vi "Register.vi"(0 "WebFrontPanel":refnum<class "WebFrontPanel.lvclass">, 5 "error in (no error)":errorcluster) -> (19 "error out":errorcluster)   [LabVIEW 2014, in "FrontPanelManager.lvclass"]
doc: "Register another WebFrontPanel"
uses:
  FrontPanelManager.lvclass
  WebFrontPanel_class/WebFrontPanel.lvclass
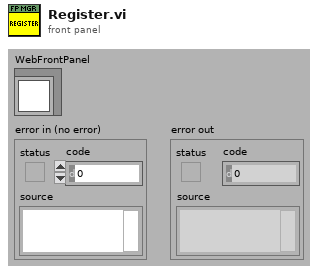
[diagram p1: front panel]
types:
  T1 = typedef "FrontPanelManager.lvclass/ObjectAttributes.ctl" = cluster{"WebFrontPanels":refnum<class "WebFrontPanel.lvclass">[], "WFP Names":string[], "Root folder":path}
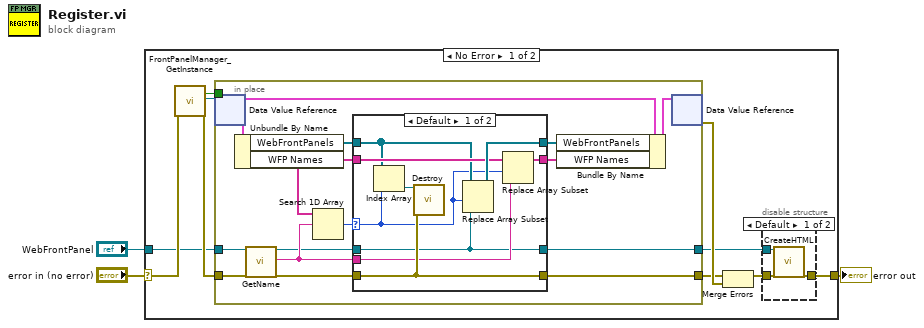
[diagram p0: block diagram]
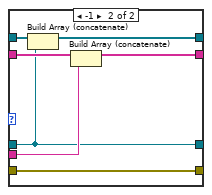
[diagram p3: hidden frame]
diagram:
  n1 = case shown="No Error" "error in (no error)" {
    selector: "error in (no error)" -> [w12 w48]
    tunnel: [w8 w48] -> w2
    tunnel: "WebFrontPanel" -> [w6 _]
    frame No Error {
      n2 = call "FrontPanelManager_GetInstance.vi"("error in (no error)"=w12) -> ("NewObjectCreated"=w4:bool, "DVRRefOut"=w7:refnum<data-value>, "error out"=w11:errorcluster)  [unwired: 14 in, 2 out]
      n3 = in-place {
        in-place-border: w6 -> [w25]
        in-place-border: w11 -> [w31]
        in-place-border: [w30] -> w10
        in-place-border: [w18] -> w5
        in-place-border: w4 -> [_]
        n4 = in-place-dvr #1(w7) -> (w22:T1)  [unwired: 1 out]
        n5 = Unbundle By Name(w22) -> ("WebFrontPanels"=w28:refnum<class "WebFrontPanel.lvclass">[], "WFP Names"=w24:string[])
        n6 = call-dynamic "GetName.vi"("reference in"=w25, "error in (no error)"=w31) -> ("reference out"=w19:refnum<class "WebFrontPanel.lvclass">, "WFP Name"=w20:string, "error out"=w29:errorcluster)  [unwired: 15 in]
        n7 = Search 1D Array(1D array=w24, element=w20) -> (index of element=w26:i32)  [unwired: 1 in]
        n8 = case shown="Default" w26 {
          selector: w26 -> [w34 _]
          tunnel: w28 -> [w35 w46]
          tunnel: w19 -> [w32 w41]
          tunnel: w24 -> [w38 w44]
          tunnel: [w39 w45] -> w27
          tunnel: [w37 w43] -> w23
          tunnel: w20 -> [w36 w42]
          tunnel: w29 -> [w40 w47]
          tunnel: [w40 w47] -> w30
          tunnel: [w32 w41] -> w18
          frame Default {
            n9 = Index Array(array=w35, index=w34) -> (element=w33:refnum<class "WebFrontPanel.lvclass">)
            n10 = call-dynamic "Destroy.vi"("reference in"=w33, "error in (no error)"=w40) -> ()  [unwired: 16 in, 2 out]
            n11 = Replace Array Subset(array=w35, new element=w32, index=w34) -> (w39:refnum<class "WebFrontPanel.lvclass">[])
            n12 = Replace Array Subset(array=w38, new element=w36, index=w34) -> (w37:string[])
          }
          frame -1 {
            n13 = Build Array (concatenate)(w46, w41) -> (w45:refnum<class "WebFrontPanel.lvclass">[])
            n14 = Build Array (concatenate)(w44, w42) -> (w43:string[])
          }
        }
        n15 = Bundle By Name(cluster=w22, "WebFrontPanels"=w27, "WFP Names"=w23) -> (w21:T1)
        n16 = in-place-dvr #1(w21) -> (w13:errorcluster)  [unwired: 1 out]
      }
      n17 = Merge Errors(w10, w13) -> (w9:errorcluster)
      n18 = disable-structure shown="Default" {
        disable-tunnel: w9 -> [w16 w17]
        disable-tunnel: [w15 w17] -> w8
        disable-tunnel: w5 -> [w14 _]
        frame condition #0 (active) {
          n19 = call "CreateHTML.vi"("WebFrontPanel"=w14, "error in (no error)"=w16) -> ("error out"=w15:errorcluster)  [unwired: 17 in]
        }
        frame condition #1 {
        }
      }
    }
    frame Error {
    }
  }
  "error out" <- w2
